vi "VisObtainFrmWrkBroadcastEvents.vi"(8 "Error":errorcluster[](array[cluster])) -> (0 "Error":errorcluster[](array[cluster]), 3 "VisFrmWrkBroadcastEvents":T1)   [LabVIEW 2018, in "Visualization.lvlib" / "VisualizeBase.lvclass"]
uses:
  VisualizeBase.lvclass
  VisFrmWrkBroadcastEvents.ctl
  Scope/ScopeShared/clEventType.ctl
  <userlib>/NIST/NISTErrorLib/NISTErrorLib.lvlib
  Scope/ScopeShared/ScopeShared.lvlib
panel:
  # "If you want to add other Request Events, open this typedef, copy an existing event and rename it to your event name."
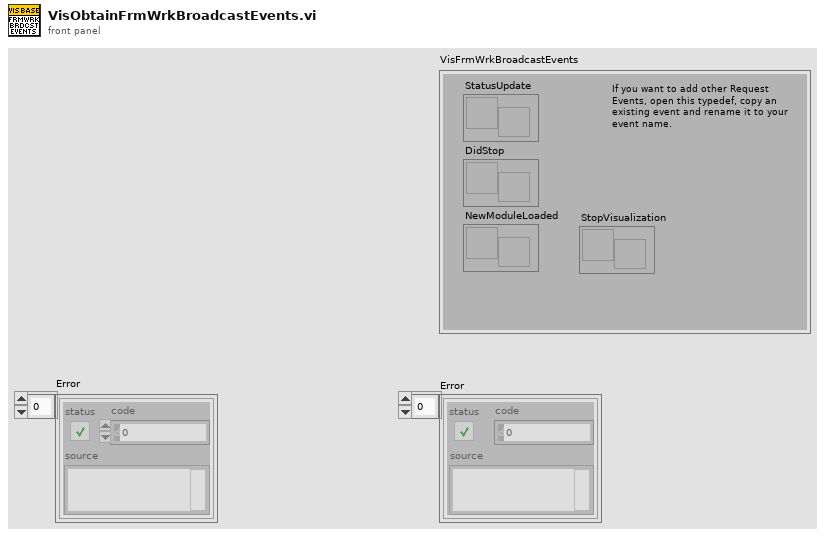
[diagram p1: front panel]
types:
  T1 = typedef "Visualization.lvlib/VisualizeBase.lvclass/VisFrmWrkBroadcastEvents.ctl" = cluster{"StatusUpdate":refnum<user-event>, "DidStop":refnum<user-event>, "NewModuleLoaded":refnum<user-event>, "StopVisualization":refnum<user-event>}
  T2 = typedef "ScopeShared.lvlib/clEventType.ctl" = cluster{"ModuleID":i32, "Data":variant}
  T3 = typedef "Visualization.lvlib/VisualizeBase.lvclass/VisRequestEvents.ctl" = cluster{"StopRequest":refnum<user-event>, "ResetRequest":refnum<user-event>, "FP Pop In or Out":refnum<user-event>}
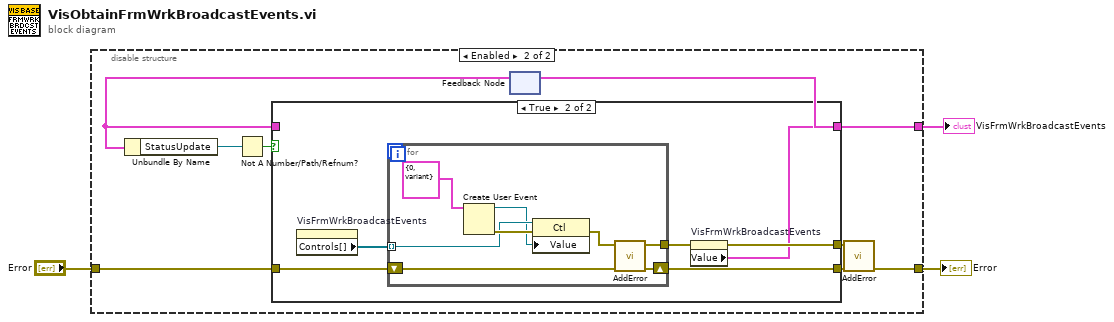
[diagram p0: block diagram]
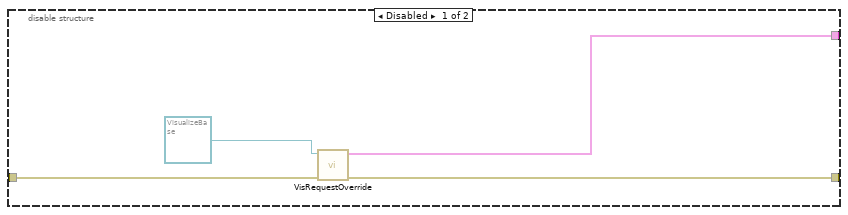
[diagram p2: hidden frame]
diagram:
  n1 = disable-structure shown="Enabled" {
    disable-tunnel: [w7 w11] -> w1
    disable-tunnel: "Error" -> [w6 w15]
    disable-tunnel: [w5 w12] -> w2
    frame Disabled {
      n2 = call-dynamic "VisRequestOverride.vi"("Error in"=w6, "Visualize"=refnum<class "VisualizeBase.lvclass"> refnum ("Visualization.lvlib:VisualizeBase_class.lvclass")) -> ("Error out"=w5:errorcluster[], "RequestEvents"=w7:T3)  [unwired: 8 in]
    }
    frame Enabled {
      n3 = feedback #1() -> (w10:T1)  [unwired: 1 in]
      n4 = Unbundle By Name(w10) -> ("StatusUpdate"=w9:refnum<user-event>)
      n5 = Not A Number/Path/Refnum?(number/path/refnum=w9) -> (NaN/Path/Refnum?=w8:bool)
      n6 = case shown="True" w8 {
        tunnel: w15 -> [w16 w23]
        tunnel: [_ w19] -> w14
        tunnel: [w16 w22] -> w13
        tunnel: [w17 w18] -> w11
        tunnel: w10 -> [w17 _]
        frame False {
        }
        frame True {
          n7 = property on="VisFrmWrkBroadcastEvents" class="Clust (strict)"() -> ("Controls[]"=w21:refnum<vi>[])  [unwired: 2 in, 2 out]
          n8 = for {
            shift-right: [w29] -> w22
            shift-left: w23 -> [w30]
            tunnel: [w28] -> w20
            tunnel: w21 -> [w26] mode=indexing
            n9 = Create User Event(user event datatype=T2 {"ModuleID"=0, "Data"=variant} ("event data")) -> (user event=w25:refnum<user-event>, error out=w31:errorcluster)  [unwired: 1 in]
            n10 = property class="Ctl"(reference=w26, error in=w31, "Value"=w25) -> (error out=w27:errorcluster)  [unwired: 1 out]
            n11 = call <userlib>:"AddError.vi"("ErrorArray In"=w30, "error in (no error)"=w27) -> ("ErrorArray Out"=w29:errorcluster[], "error out"=w28:errorcluster)  [unwired: 8 in]
          }
          n12 = property on="VisFrmWrkBroadcastEvents" class="Clust (strict)"(error in=w20) -> (error out=w19:errorcluster, "Value"=w18:T1)  [unwired: 1 in, 1 out]
        }
      }
      n13 = feedback-in #1(w11) -> ()
      n14 = call <userlib>:"AddError.vi"("ErrorArray In"=w13, "error in (no error)"=w14) -> ("ErrorArray Out"=w12:errorcluster[])  [unwired: 8 in, 1 out]
    }
  }
  "VisFrmWrkBroadcastEvents" <- w1
  "Error" <- w2
